vi "Host_Data_Acquisition.vi"() -> ()   [LabVIEW 2018]
uses:
  <vilib>/Platform/TimedLoop/XDataNode/timing_clust.ctl
  <vilib>/Platform/TimedLoop/XDataNode/nitl_modes.ctl
  <vilib>/Platform/TimedLoop/XDataNode/wakeup.ctl
  <vilib>/Platform/TimedLoop/XDataNode/XDataNode.xnode
  <vilib>/Platform/TimedLoop/XDataNode/XDNodeRunTimeDep.lvlib
panel:
  in  "Collect Data":bool
  in  "index":i32
  out "Data of Channel #":dbl(graph)
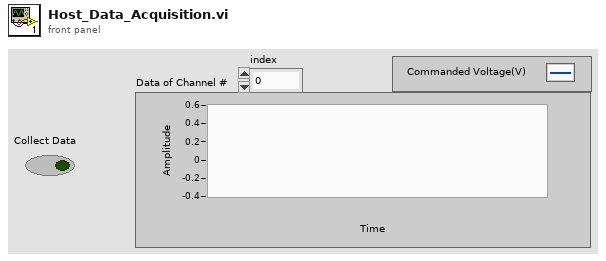
[diagram p1: front panel]
types:
  T1 = enum16{"open", "open or create", "create or replace", "create", "open (read-only)"}
  T2 = typedef "XDNodeRunTimeDep.lvlib/timing_clust.ctl" = cluster{"Expected End [f-1]":u64, "Actual End [f-1]":u64, "Finished Late? [f-1]":bool, "Expected End [i-1]":u64, "Actual End [i-1]":u64, "Finished Late? [i-1]":bool, "Expected Start [i]":u64, "Actual Start [i]":u64, "Expected Start [f]":u64, "Actual Start [f]":u64, "Source Name":string, "Structure Name":string, "Period":i64, "Deadline":i64, "Offset":i64, "Start":i64, "Priority":i32, "Timeout":i32, "Mode":T3, "Wakeup Reason":T4, "Error":errorcluster, "Source Type":string, "Secondary Source Type":string, "Global End Time":u64, "Global Start Time":u64, "Frame Duration":u64, "Iteration Duration":u64, "Assigned CPU":i32, "I/O Scan Engine Mode":u32}
  T3 = typedef "XDNodeRunTimeDep.lvlib/nitl_modes.ctl" = enum32{"No Change", "Process missed periods, maintain original phase", "Discard missed periods, maintain original phase", "Process missed periods, ignore original phase", "Discard missed periods, ignore original phase"}
  T4 = typedef "XDNodeRunTimeDep.lvlib/wakeup.ctl" = enum32{"Normal", "Aborted", "Asynchronous wakeup", "Timing source error", "Timed loop error", "Timeout"}
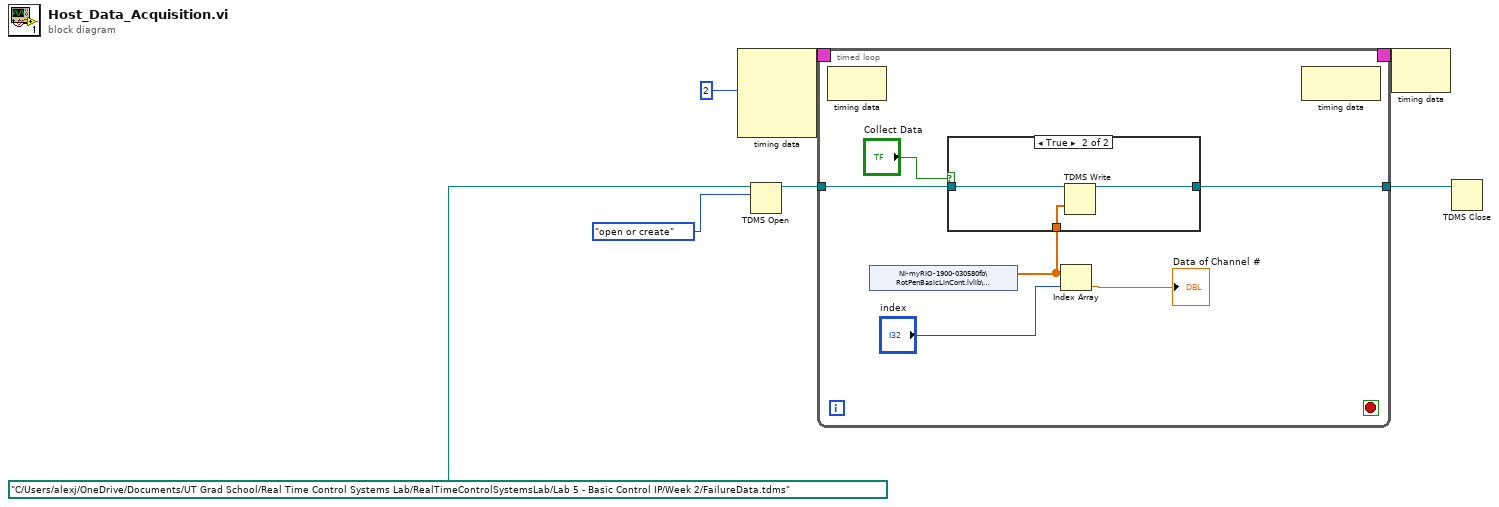
[diagram p0: block diagram]
diagram:
  n1 = node-c288(i64 2 ("Period")) -> (w7:T2)  [unwired: 3 in]
  n2 = TDMS Open(10:T1."open or create" ("operation (0:open)"), 11:path "C:/Users/alexj/OneDrive/Documents/UT Grad School/Real Time Control Systems Lab/RealTimeControlSystemsLab/Lab 5 - Basic Control IP/Week 2/FailureData.tdms" ("file path")) -> (3:w4:refnum<k34>)  [unwired: 5 in, 1 out]
  n3 = timed-loop {
    timing: w7 -> [_]
    timing-out: [_] -> w6
    tunnel: w4 -> [w11]
    tunnel: [w10] -> w3
    stop <- _ stop-if-true
    n4 = node-c288() -> ()  [unwired: 1 in, 1 out]
    n5 = shared-variable "NI-myRIO-1900-030580fb\\RotPenBasicLinCont.lvlib\\UltraMechaVariable"() -> (w9:dbl[])  [unwired: 1 in, 1 out]
    n6 = case shown="True" "Collect Data" {
      tunnel: w11 -> [w14 w17]
      tunnel: [w14 w16] -> w10
      tunnel: w9 -> [_ w15]
      frame False {
      }
      frame True {
        n7 = TDMS Write(0:w17, 9:w15) -> (4:w16:refnum<k34>)  [unwired: 4 in, 3 out]
      }
    }
    n8 = Index Array(array=w9, index="index") -> (element=→"Data of Channel #":dbl)
    n9 = node-c288() -> ()  [unwired: 1 in, 1 out]
  }
  n10 = node-c288(w6) -> ()  [unwired: 1 out]
  n11 = TDMS Close(11:w3) -> ()  [unwired: 1 in, 2 out]
